vi "Remove Property.vi"(8 "error in (no error)":errorcluster caption="错误输入（无错误）", 10 "Property Name":string, 11 "Item输入":refnum<class "Item.lvclass">) -> (0 "error out":errorcluster caption="错误输出", 2 "removed":bool, 3 "Item输出":refnum<class "Item.lvclass">)   [LabVIEW 2013, in "Hierarchy Framework.lvlib" / "Item.lvclass"]
doc: "Removes the property specified by <B>Property Name</B> from a custom device item."
uses:
  Item.lvclass
  Item.lvclass/Item.ctl
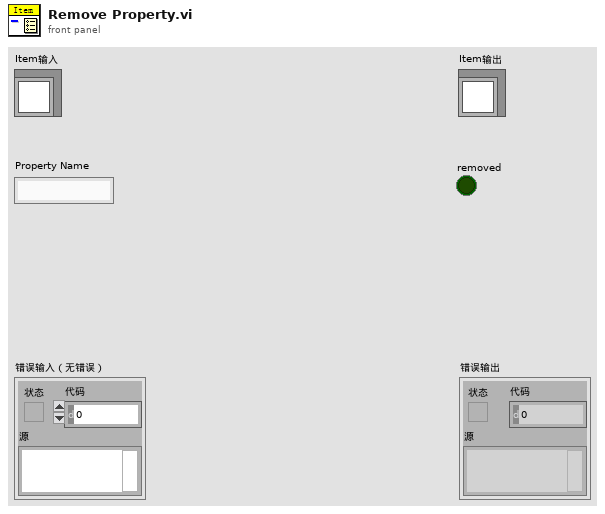
[diagram p1: front panel]
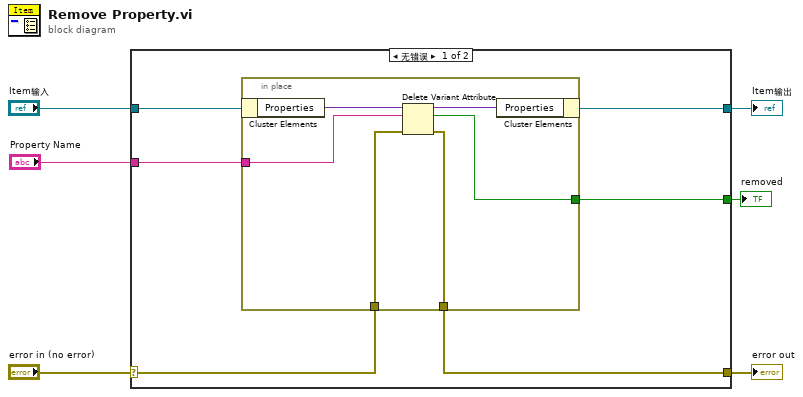
[diagram p0: block diagram]
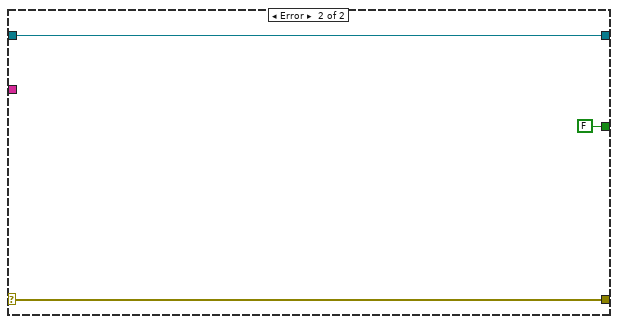
[diagram p2: hidden frame]
diagram:
  n1 = case shown="无错误" "error in (no error)" {
    selector: "error in (no error)" -> [w8 w21]
    tunnel: [w7 w21] -> w5
    tunnel: [w11 w20] -> w3
    tunnel: "Item输入" -> [w12 w20]
    tunnel: [w10 FALSE ("replaced")] -> w1
    tunnel: "Property Name" -> [w9 _]
    frame No Error {
      n2 = in-place {
        in-place-border: [w17] -> w10
        in-place-border: w9 -> [w13]
        in-place-border: w8 -> [w16]
        in-place-border: [w15] -> w7
        n3 = in-place-cluster #1(w12) -> ("Properties"=w14:variant)
        n4 = Delete Variant Attribute(4:w16, 6:w13, 7:w14) -> (0:w15:errorcluster, 2:w17:bool, 3:w18:variant)
        n5 = in-place-cluster #1("Properties"=w18) -> (w11:refnum<class "Item.lvclass">)
      }
    }
    frame Error {
    }
  }
  "error out" <- w5
  "Item输出" <- w3
  "removed" <- w1
